vi "Configure Temperature.vi"(6 "NPLC":dbl=1.0, 7 "Aperture Seconds":dbl, 8 "error in (no error)":errorcluster, 9 "Transducer Type":u16(ring)=1 items=["Thermocouple", "Thermistor", "3-wire RTD", " 4-wire RTD"], 10 "Set Aperture or NPLC":bool=TRUE, 11 "VISA resource name":refnum<visa-resource-name>) -> (0 "error out":errorcluster, 3 "VISA resource name out":refnum<visa-resource-name>)   [LabVIEW 2021, in "Keithley DMM7510.lvlib"]
doc: "This VI configures the Temperature measurement function parameters like transducer type, NPLC and the aperture setting."
uses:
  Keithley DMM7510.lvlib
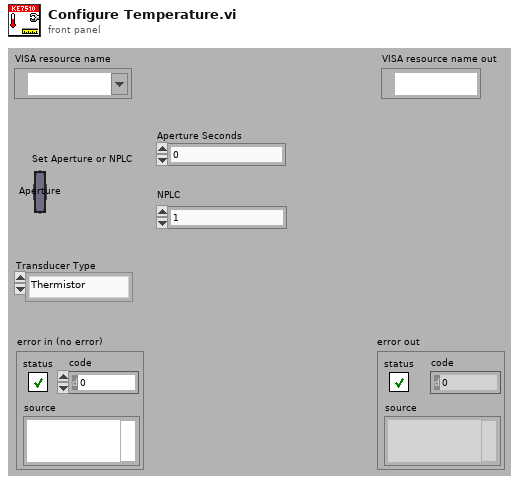
[diagram p1: front panel]
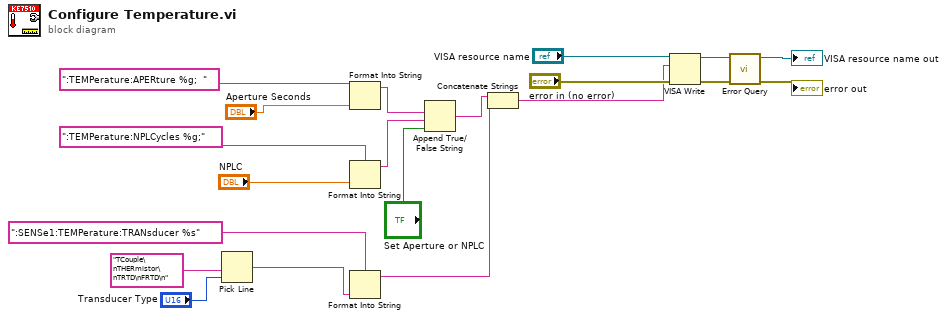
[diagram p0: block diagram]
diagram:
  n1 = Pick Line(multi-line string="TCouple\nTHERmistor\nTRTD\nFRTD\n", line index="Transducer Type") -> (output string=w13:string)  [unwired: 1 in]
  n2 = Format Into String(format string=":TEMPerature:APERture %g;  ", "Aperture Seconds") -> (resulting string=w2:string)  [unwired: 2 in, 1 out]
  n3 = Format Into String(format string=":TEMPerature:NPLCycles %g;", "NPLC") -> (resulting string=w3:string)  [unwired: 2 in, 1 out]
  n4 = Format Into String(format string=":SENSe1:TEMPerature:TRANsducer %s", w13) -> (resulting string=w11:string)  [unwired: 2 in, 1 out]
  n5 = Append True/False String(1:"Set Aperture or NPLC", 2:w3, 3:w2) -> (0:w1:string)  [unwired: 1 in]
  n6 = Concatenate Strings(w1, w11) -> (w16:string)
  n7 = VISA Write(VISA resource name="VISA resource name", write buffer=w16, error in (no error)="error in (no error)") -> (VISA resource name out=w10:refnum<visa-resource-name>, error out=w9:errorcluster)  [unwired: 1 out]
  n8 = call "Error Query.vi"("error in (no error)"=w9, "VISA resource name"=w10) -> ("error out"=→"error out":errorcluster, "VISA resource name out"=→"VISA resource name out":refnum<visa-resource-name>)  [unwired: 6 in, 2 out]
